vi "Arm.vi"(11 "Console Reference":refnum<vi>) -> ()   [LabVIEW 2020]
uses:
  <vilib>/Utility/file.llb/Write Delimited Spreadsheet (DBL).vi
panel:
  in  "start":bool
  in  "Save":bool
  in  "python":string
  in  "Send":bool
  in  "Clear":bool
  in  "Tab Control":T1(tab)=enum."Picture"
  out "Graph":dbl[][](graph)
  out "XY Plot":cluster{dbl[], dbl[]}[](graph)
  out "2D":picture
  out "3D":refnum<vi>(3d-picture)
  out "Gauge":dbl[](array[knob]) scale=-100.0..100.0
  out "Last Line":string
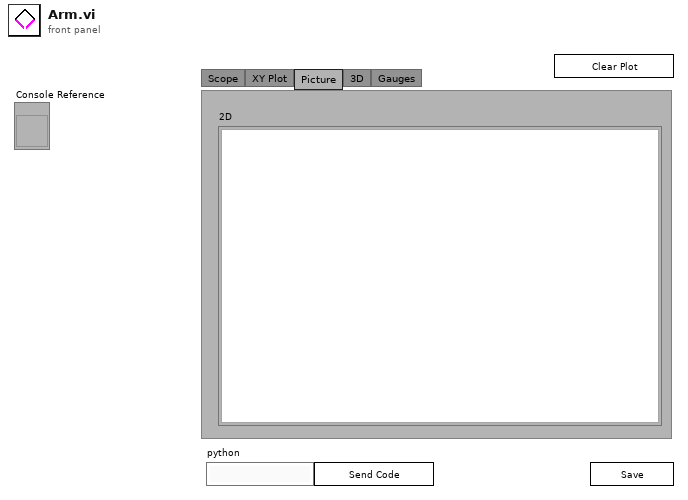
[diagram p1: front panel]
types:
  T1 = enum32{"Scope", "XY Plot", "Picture", "3D", "Gauges"}
  T2 = enum16{"Not data", "single values", "XY pairs", "Arrays"}
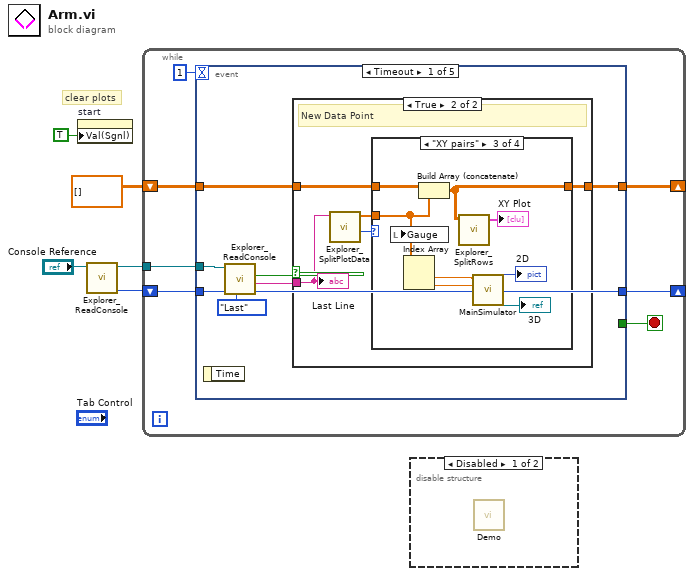
[diagram p0: block diagram]
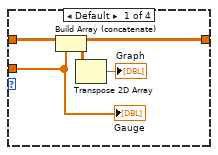
[diagram p4: hidden frame]
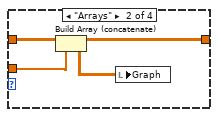
[diagram p5: hidden frame]
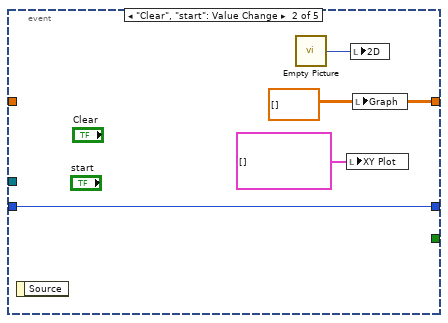
[diagram p7: hidden frame]
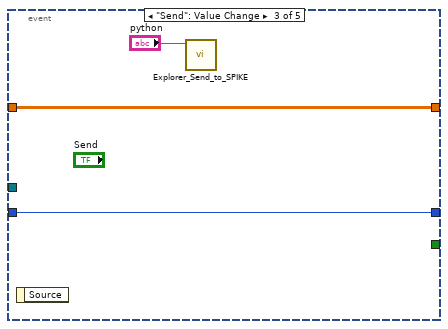
[diagram p8: hidden frame]
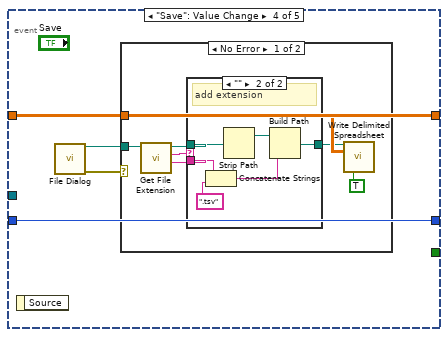
[diagram p9: hidden frame]
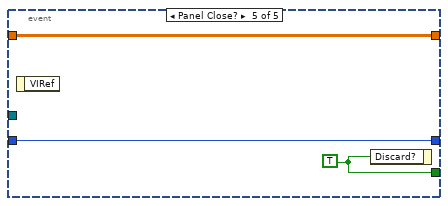
[diagram p12: hidden frame]
diagram:
  # "clear plots"
  n1 = property on="start" class="Bool (strict)"("Val(Sgnl)"=TRUE ("Value (Signaling)")) -> ()  [unwired: 2 in, 2 out]
  n2 = call "Explorer_ReadConsole.vi"("String in"="Console Reference") -> ("index out"=w4:i32, "String out"=w3:refnum<vi>)  [unwired: 7 in, 2 out]
  n3 = while {
    shift-right: [w10] -> _
    shift-left: w4 -> [w9]
    shift-right: [w7] -> _
    shift-left: dbl[][] [] -> [w8]
    tunnel: w3 -> [w6]
    stop <- w11 stop-if-true
    n4 = event shown="[0] Timeout" {
      selector: _ -> [_ _ _ _ _]
      dyn-events: _ -> [_ _ _ _ _]
      timeout: 1 -> [_ _ _ _ _]
      tunnel: [_ _ _ _ w70] -> w11
      tunnel: [w17 w46 w48 w53 w69] -> w10
      tunnel: w9 -> [w18 w46 w48 w53 w69]
      tunnel: w8 -> [w20 _ w49 w52 w68]
      tunnel: [w19 w45 w49 w52 w68] -> w7
      tunnel: w6 -> [w14 _ _ _ _]
      event Timeout {
        n5 = event-data() -> ()  [unwired: 1 in, 1 out]
        n6 = call "Explorer_ReadConsole.vi"("Reading"=enum16{"Next", "Last"}."Last" ("type"), "index in"=w18, "String in"=w14) -> ("index out"=w17:i32, "New Line"=w16:string, "New point?"=w15:bool)  [unwired: 5 in, 1 out]
        n7 = case shown="True" w15 {
          tunnel: w16 -> [_ w26]
          tunnel: w20 -> [w21 w25]
          tunnel: [w21 w24] -> w19
          frame False {
            # "nothing new"
          }
          frame True {
            # "New Data Point"
            n8 = call "Explorer_SplitPlotData.vi"("Value"=w26) -> ("Data type"=w23:T2, "Array"=w22:dbl[])  [unwired: 9 in]
            n9 = case shown="\"XY pairs\"" w23 {
              tunnel: w25 -> [w30 w33 w41 w42]
              tunnel: [w29 w31 w40 w42] -> w24
              tunnel: w22 -> [w27 w32 w36 _]
              frame Default {
                n10 = Build Array (concatenate)(w30, w27) -> (w29:dbl[][])
                n11 = Transpose 2D Array(2D array=w29) -> (transposed array=→"Graph":dbl[][])
                "Gauge" <- w27
              }
              frame "Arrays" {
                n12 = Build Array (concatenate)(w33, w32) -> (w31:dbl[][])
                n13 = local write "Graph"(w31) -> ()
              }
              frame "XY pairs" {
                n14 = local write "Gauge"(w36) -> ()
                n15 = Index Array(array=w36) -> (element #1=w35:dbl, element #2=w34:dbl)  [unwired: 2 in]
                n16 = Build Array (concatenate)(w41, w36) -> (w40:dbl[][])
                n17 = call "Explorer_SplitRows.vi"("Array in"=w40) -> ("XY Plot"=→"XY Plot":cluster{dbl[], dbl[]}[])  [unwired: 10 in]
                n18 = call "MainSimulator.vi"("beta 2"=w34, "beta 1"=w35) -> ("3D Picture"=→"3D":refnum<vi>, "Canvas"=→"2D":picture)  [unwired: 8 in]
              }
              frame "Not data" {
              }
            }
            "Last Line" <- w26
          }
        }
      }
      event "Clear", "start": Value Change {
        w45 = dbl[][] []
        n19 = event-data() -> ()  [unwired: 1 in, 1 out]
        n20 = call "Empty Picture"() -> ("empty picture"=w43:picture)
        n21 = local write "XY Plot"(cluster{dbl[], dbl[]}[] [] ("XY Plot")) -> ()
        n22 = local write "2D"(w43) -> ()
        n23 = local write "Graph"(w45) -> ()
      }
      event "Send": Value Change {
        n24 = event-data() -> ()  [unwired: 1 in, 1 out]
        n25 = call "Explorer_Send_to_SPIKE.vi"("python"="python") -> ()  [unwired: 11 in]
      }
      event "Save": Value Change {
        n26 = event-data() -> ()  [unwired: 1 in, 1 out]
        n27 = call "File Dialog"() -> ("selected path"=w51:path, "error out"=w50:errorcluster)  [unwired: 12 in, 2 out]
        n28 = case shown="No Error" w50 {
          tunnel: w52 -> [w60 _]
          tunnel: w51 -> [w58 _]
          frame No Error {
            n29 = call <vilib>:"Get File Extension.vi"("file"=w58) -> ("filename without extension"=w54:string, "lowercase file extension"=w57:string, "dup file"=w55:path)  [unwired: 6 in, 2 out]
            n30 = case shown="\"\"" w57 {
              tunnel: [w61 w63] -> w56
              tunnel: w55 -> [w61 w65]
              tunnel: w54 -> [_ w67]
              frame Default {
              }
              frame "" {
                # "add extension"
                n31 = Concatenate Strings(w67, ".tsv" ("pattern (all files)")) -> (w62:string)
                n32 = Strip Path(path=w65) -> (stripped path=w64:path)  [unwired: 1 out]
                n33 = Build Path(base path=w64, name or relative path=w62) -> (appended path=w63:path)
              }
            }
            n34 = call-poly <vilib>:"Write Delimited Spreadsheet.vi"("file path (dialog if empty)"=w56, "2D data"=w60, "transpose? (no:F)"=TRUE) -> ()  [unwired: 11 in, 2 out]
          }
          frame Error {
          }
        }
      }
      event Panel Close? {
        w70 = TRUE ("Discard?")
        n35 = event-data() -> ()  [unwired: 1 in, 1 out]
        n36 = event-data("Discard?"=w70) -> ()  [unwired: 1 in, 1 out]
      }
    }
  }
  n37 = disable-structure shown="Disabled" {
    frame Disabled {
      n38 = call "Demo.vi"() -> ()  [unwired: 12 in]
    }
    frame Enabled {
    }
  }
